vi "Ballard 1553 - Initialize.vi"(7 "RT Config Filepath":path, 8 "Error (in)":errorcluster, 9 "Compiled.Settings":T1 {"channels"."RTs"."Mode Codes"."Timestamp Channel Data Reference" format="%.0x"; "channels"."RTs"."subAddresses"."Timestamp Channel Data Reference" format="%.0x"; "channels"."RTs"."Status Channel Data Reference" format="%.0x"; "channels"."RTs"."Command Channels Refs" format="%.0x"; "channels"."BC"."Acyclic Frames Trigger Channels Refs" format="%.0x"; "channels"."BC"."Command Channels Refs" format="%.0x"; "channels"."BC"."messages"."Timestamp Channel Data Reference" format="%.0x"; "channels"."BC"."messages"."Status Channel Data Refs" format="%.0x"; "channels"."BC"."messages"."Words Item Refs" format="%.0x"}, 11 "Card Parameters (in)":T16) -> (0 "Error (out)":errorcluster, 3 "Card Parameters (out)":T16)   [LabVIEW 2019, in "Ballard MIL-1553 Engine.lvlib"]
doc: "Arinc-429 Board Initialization."
uses:
  Ballard MIL-1553 Engine.lvlib
  Controls/Card Parameters.ctl
  Shared/Controls and Global/Initialization Method.ctl
  Shared/Controls and Global/Compiled.Settings.ctl
  Shared/Controls and Global/RT Channel.ctl
  Shared/Controls and Global/RT BC.ctl
  <vilib>/NI VeriStand/Custom Device API/Custom Device Item Ref.ctl
  Shared/Controls and Global/RT Message.ctl
  Shared/Controls and Global/RT messageType.ctl
  Shared/Controls and Global/RT CWD1.ctl
  Shared/Controls and Global/RT CWD2.ctl
  <vilib>/NI VeriStand/Custom Device API/Data Reference.ctl
  <vilib>/NI VeriStand/Custom Device API/Block Data Reference.ctl
  Shared/Controls and Global/RT Remote Terminal.ctl
  Shared/Controls and Global/RT Remote Terminal_rtMode.ctl
  Shared/Controls and Global/RT Remote Terminal_RT subAddress.ctl
  Shared/Controls and Global/RT Remote Terminal_RT direction.ctl
  Shared/Controls and Global/RT Remote Terminal_RT Mode Code.ctl
  <instrlib>/BTICardLib/Private/Initialize By Card Number and Core Number.vi
  <instrlib>/BTICardLib/Private/Initialize By Slot Number and Core Number.vi
  <instrlib>/BTICardLib/Private/IO/Action-Status/Write External LED.vi
  <instrlib>/BTICardLib/Private/Configure All From XML.vi
  <instrlib>/BTI1553Lib/Private/Channel/Configure/Configure All From XML.vi
  <instrlib>/BTICardLib/BTICardLV.lvlib
  Shared/Ballard 1553 Shared.lvlib
  <instrlib>/BTI1553Lib/BTI1553LV.lvlib
  <vilib>/NI VeriStand/Custom Device Tools/Custom Device Utility Library/Custom Device Utility Library.lvlib
  <vilib>/NI VeriStand/Custom Device API/Custom Device API.lvlib
panel:
  out "Card Type":string
  out "Product String":string
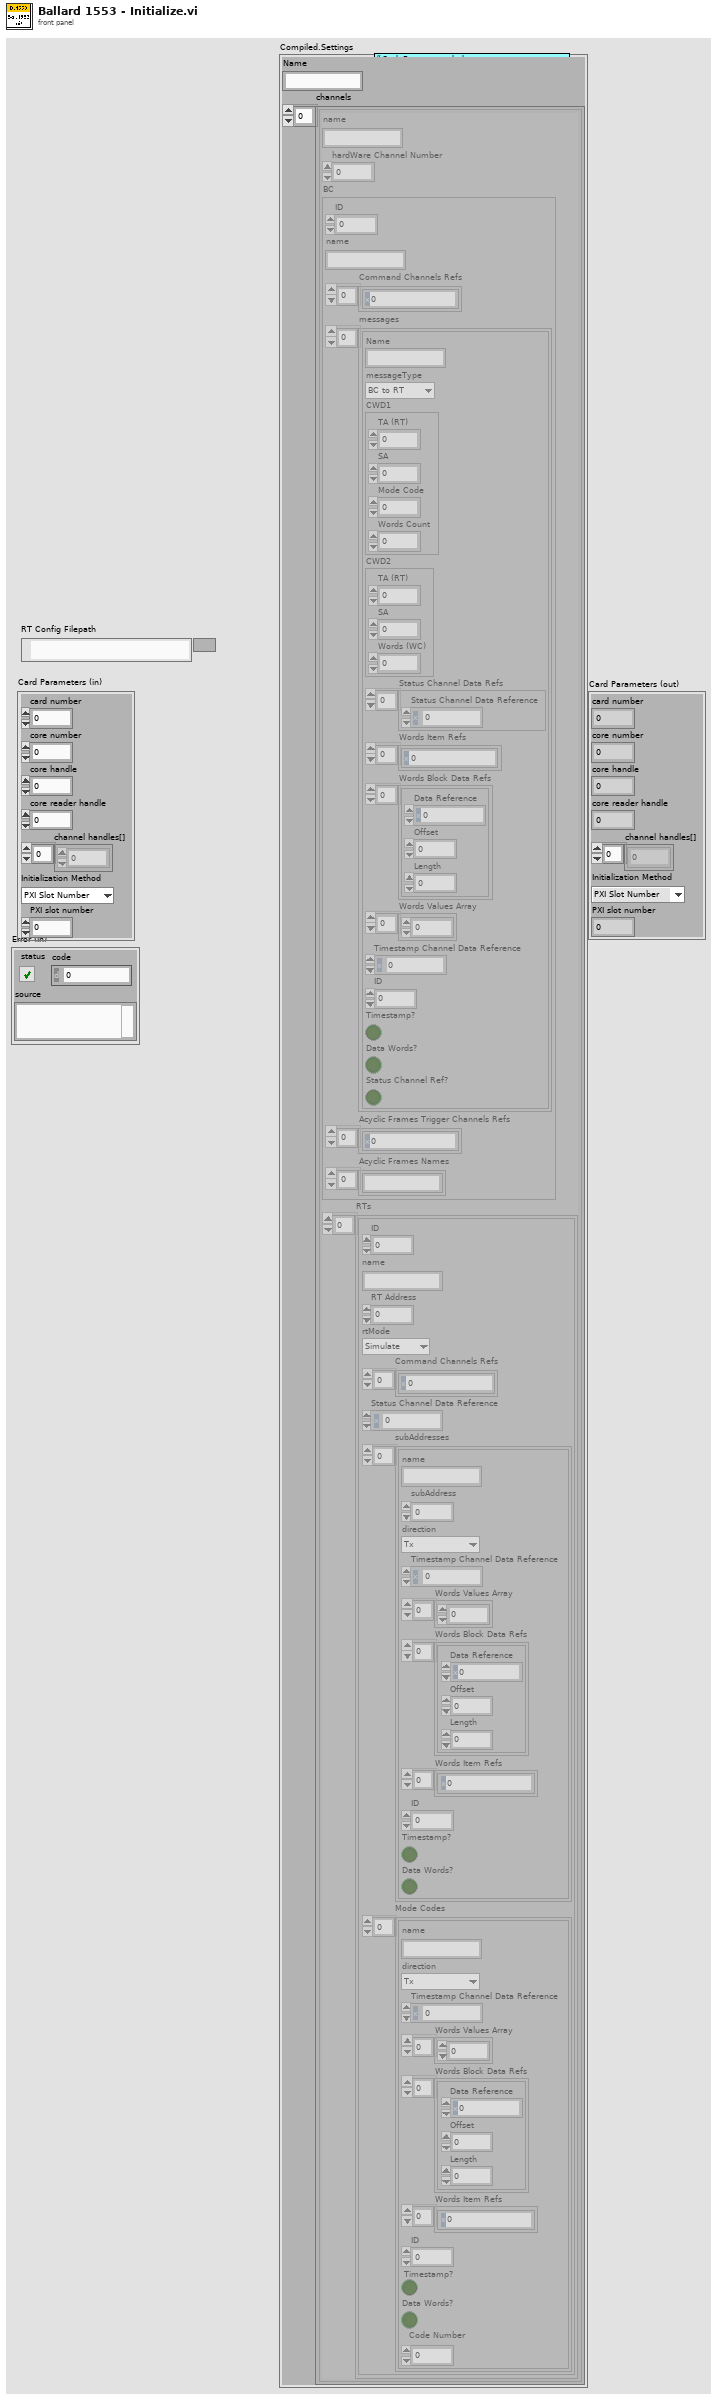
[diagram p1: front panel]
types:
  T1 = typedef "Ballard 1553 Shared.lvlib/Compiled.Settings.ctl" = cluster{"Name":string, "channels":T2[]}
  T2 = typedef "Ballard 1553 Shared.lvlib/RT Channel.ctl" = cluster{"name":string, "hardWare Channel Number":u16, "BC":T3, "RTs":T11[]}
  T3 = typedef "Ballard 1553 Shared.lvlib/RT BC.ctl" = cluster{"ID":i32, "name":string, "Command Channels Refs":T4[], "messages":T5[], "Acyclic Frames Trigger Channels Refs":T4[], "Acyclic Frames Names":string[]}
  T4 = typedef "Custom Device API.lvlib/Custom Device Item Ref.ctl" = u64
  T5 = typedef "Ballard 1553 Shared.lvlib/RT Message.ctl" = cluster{"Name":string, "messageType":T6, "CWD1":T7, "CWD2":T8, "Status Channel Data Refs":T9[], "Words Item Refs":T4[], "Words Block Data Refs":T10[], "Words Values Array":u16[], "Timestamp Channel Data Reference":T9, "ID":i32, "Timestamp?":bool, "Data Words?":bool, "Status Channel Ref?":bool}
  T6 = typedef "Ballard 1553 Shared.lvlib/RT messageType.ctl" = enum16{"BC to RT", "RT to BC", "RT to RT", "MC (Rx)", "MC (Tx)"}
  T7 = typedef "Ballard 1553 Shared.lvlib/RT CWD1.ctl" = cluster{"TA (RT)":i8, "SA":i8, "Mode Code":i8, "Words Count":i8}
  T8 = typedef "Ballard 1553 Shared.lvlib/RT CWD2.ctl" = cluster{"TA (RT)":i8, "SA":i8, "Words (WC)":i8}
  T9 = typedef "Custom Device API.lvlib/Data Reference.ctl" = i32
  T10 = typedef "Custom Device API.lvlib/Block Data Reference.ctl" = cluster{"Data Reference":T9, "Offset":u64, "Length":u64}
  T11 = typedef "Ballard 1553 Shared.lvlib/RT Remote Terminal.ctl" = cluster{"ID":i32, "name":string, "RT Address":i32, "rtMode":T12, "Command Channels Refs":T4[], "Status Channel Data Reference":T9, "subAddresses":T13[], "Mode Codes":T15[]}
  T12 = typedef "Ballard 1553 Shared.lvlib/RT Remote Terminal_rtMode.ctl" = enum16{"Simulate", "Monitor", "Disable"}
  T13 = typedef "Ballard 1553 Shared.lvlib/RT Remote Terminal_RT subAddress.ctl" = cluster{"name":string, "subAddress":i8, "direction":T14, "Timestamp Channel Data Reference":T9, "Words Values Array":u16[], "Words Block Data Refs":T10[], "Words Item Refs":T4[], "ID":i32, "Timestamp?":bool, "Data Words?":bool}
  T14 = typedef "Ballard 1553 Shared.lvlib/RT Remote Terminal_RT direction.ctl" = enum16{"Tx", "Rx"}
  T15 = typedef "Ballard 1553 Shared.lvlib/RT Remote Terminal_RT Mode Code.ctl" = cluster{"name":string, "direction":T14, "Timestamp Channel Data Reference":T9, "Words Values Array":u16[], "Words Block Data Refs":T10[], "Words Item Refs":T4[], "ID":i32, "Timestamp?":bool, "Data Words?":bool, "Code Number":i32}
  T16 = typedef "Ballard MIL-1553 Engine.lvlib/Card Parameters.ctl" = cluster{"card number":i32, "core number":i32, "core handle":u64, "core reader handle":u64, "channel handles[]":u64[], "Initialization Method":T17, "PXI slot number":i32}
  T17 = typedef "Ballard 1553 Shared.lvlib/Initialization Method.ctl" = enum16{"PXI Slot Number", "Card Number"}
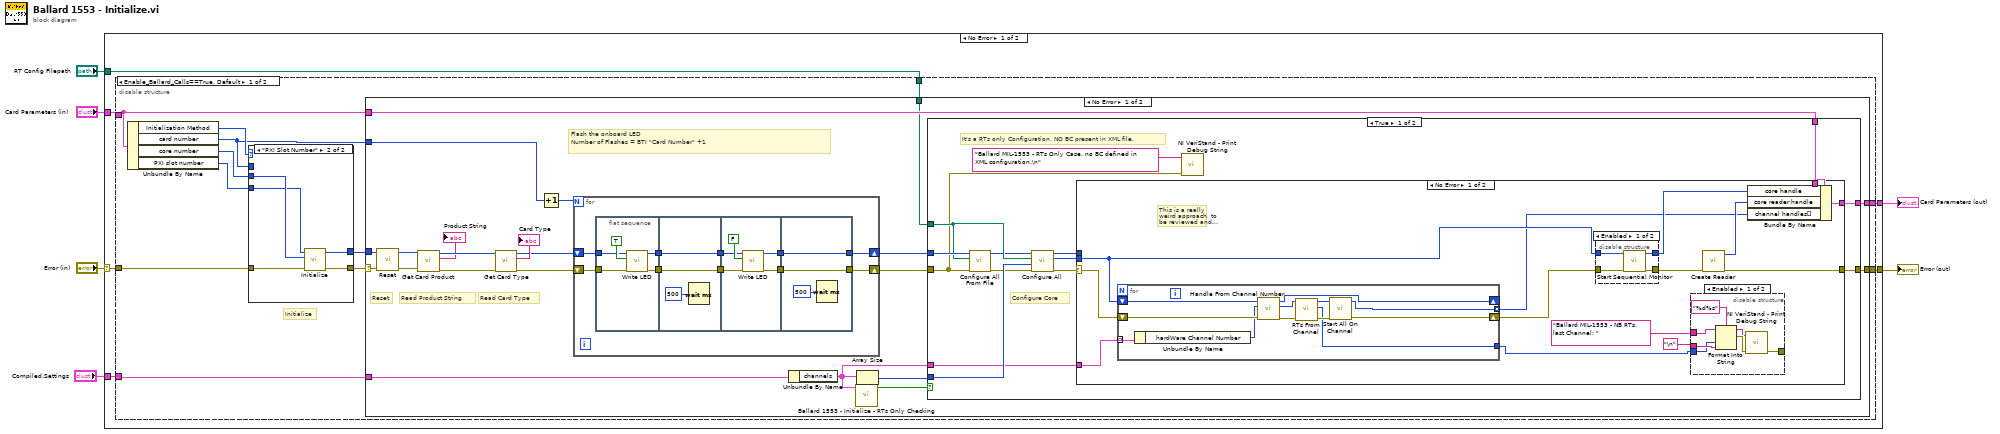
[diagram p0: block diagram]
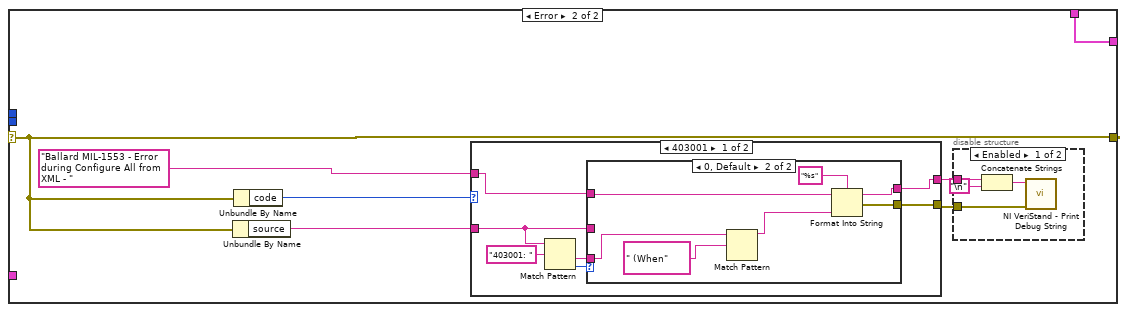
[diagram p4: hidden frame]
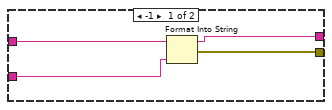
[diagram p6: hidden frame]
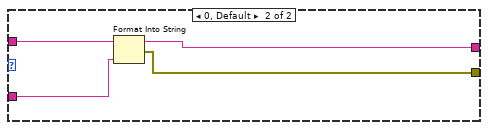
[diagram p7: hidden frame]
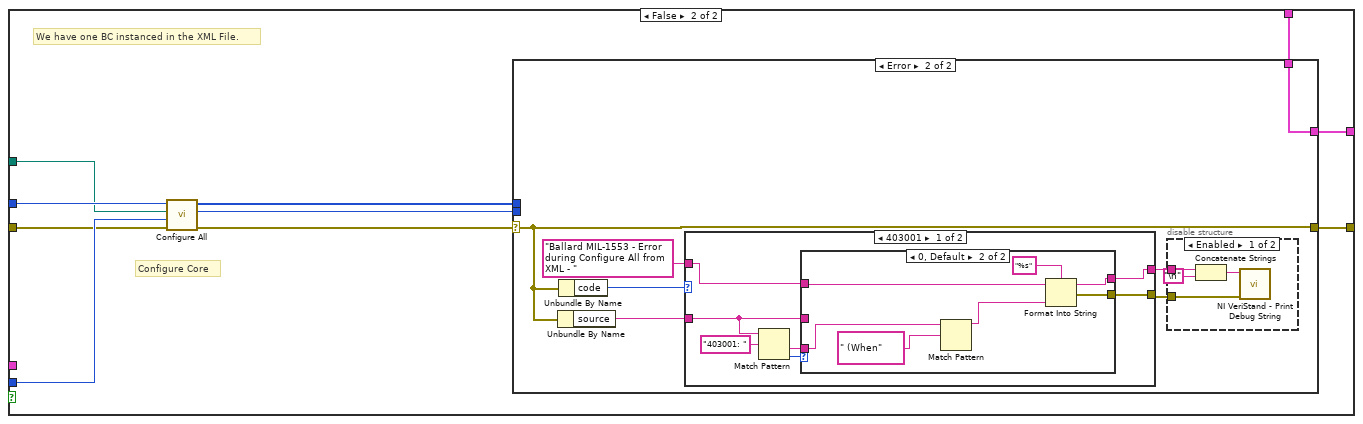
[diagram p8: hidden frame]
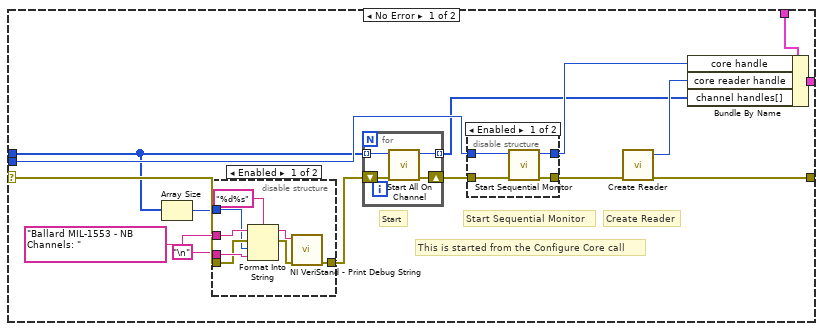
[diagram p9: hidden frame]
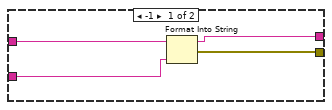
[diagram p13: hidden frame]
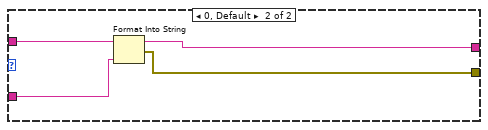
[diagram p14: hidden frame]
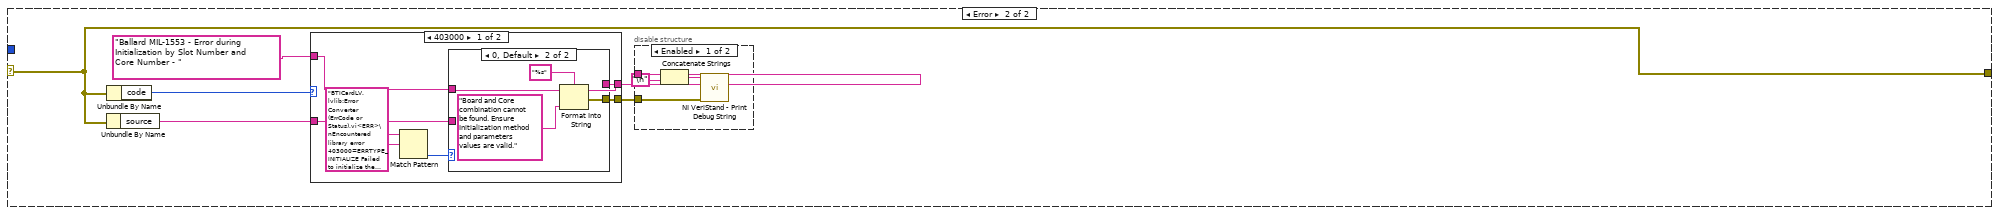
[diagram p15: hidden frame]
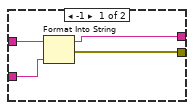
[diagram p17: hidden frame]
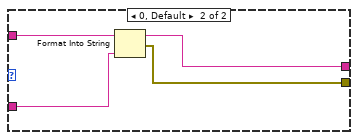
[diagram p18: hidden frame]
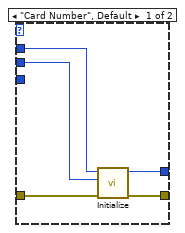
[diagram p19: hidden frame]
diagram:
  n1 = case shown="No Error" "Error (in)" {
    selector: "Error (in)" -> [w9 w279]
    tunnel: [w12 T16 {"card number"=0, "core number"=0, "core handle"=0, "core reader handle"=0, "channel handles[]"=[], "Initialization Method"=enum."PXI Slot Number", "PXI slot number"=0} ("Card Parameters (in)")] -> w6
    tunnel: "RT Config Filepath" -> [w11 _]
    tunnel: [w10 w279] -> w4
    tunnel: "Card Parameters (in)" -> [w8 _]
    tunnel: "Compiled.Settings" -> [w7 _]
    frame No Error {
      n2 = disable-structure shown="Enable_Ballard_Calls==True, Default" {
        disable-tunnel: [w23 w276] -> w12
        disable-tunnel: w11 -> [w15 _]
        disable-tunnel: [w14 w277] -> w10
        disable-tunnel: w9 -> [w22 w277]
        disable-tunnel: w8 -> [w21 w276]
        disable-tunnel: w7 -> [w16 _]
        frame condition #0 (active) {
          # "Initialize"
          n3 = Unbundle By Name(w21) -> ("Initialization Method"=w20:T17, "card number"=w19:i32, "core number"=w18:i32, "PXI slot number"=w17:i32)
          n4 = case shown="\"PXI Slot Number\"" w20 {
            tunnel: [w270 w275] -> w24
            tunnel: [w269 w274] -> w13
            tunnel: w19 -> [w268 _]
            tunnel: w22 -> [w267 w273]
            tunnel: w18 -> [w266 w272]
            tunnel: w17 -> [_ w271]
            frame "Card Number", Default {
              n5 = call-poly <instrlib>:"Initialize.vi"("error in (no error)"=w267, "core number"=w266, "card number"=w268) -> ("error out"=w269:errorcluster, "core handle out"=w270:u64)  [unwired: 7 in]
            }
            frame "PXI Slot Number" {
              n6 = call-poly <instrlib>:"Initialize.vi"("error in (no error)"=w273, "core number"=w272, "slot number"=w271) -> ("error out"=w274:errorcluster, "core handle out"=w275:u64)  [unwired: 7 in]
            }
          }
          n7 = case shown="No Error" w13 {
            selector: w13 -> [w29 w237]
            tunnel: w24 -> [w46 _]
            tunnel: [w45 _] -> w23
            tunnel: w21 -> [w35 _]
            tunnel: w19 -> [w34 _]
            tunnel: w16 -> [w33 _]
            tunnel: w15 -> [w27 _]
            tunnel: [w30 w237] -> w14
            frame No Error {
              # "Flash the onboard LED\nNumber of Flashes = BTI \"Card Number\" +1"
              # "Read Card Type"
              # "Read Product String"
              # "Reset"
              n8 = call <instrlib>:"Reset.vi"("error in (no error)"=w29, "core handle in"=w46) -> ("error out"=w39:errorcluster, "core handle out"=w40:u64)  [unwired: 8 in]
              n9 = call <instrlib>:"Get Card Product.vi"("error in (no error)"=w39, "core handle in"=w40) -> ("error out"=w43:errorcluster, "product string out"=→"Product String":string, "core handle out"=w44:u64)  [unwired: 7 in]
              n10 = call <instrlib>:"Get Card Type.vi"("error in (no error)"=w43, "core handle in"=w44) -> ("error out"=w37:errorcluster, "type string out"=→"Card Type":string, "core handle out"=w38:u64)  [unwired: 7 in]
              n11 = Increment(x=w34) -> (x+1=w36:i32)
              n12 = for {
                N: w36 -> [_]
                shift-right: [w212] -> w28
                shift-left: w38 -> [w214]
                shift-right: [w211] -> w31
                shift-left: w37 -> [w213]
                n13 = flat-sequence {
                  tunnel: [w224] -> w220
                  tunnel: [w223] -> w219
                  tunnel: w214 -> [w222]
                  tunnel: w213 -> [w221]
                  tunnel: [w227] -> w218
                  tunnel: w220 -> [w227]
                  tunnel: [w226] -> w217
                  tunnel: w219 -> [w226]
                  tunnel: w218 -> [w232]
                  tunnel: [w231] -> w216
                  tunnel: [w230] -> w215
                  tunnel: w217 -> [w229]
                  tunnel: [w235] -> w211
                  tunnel: w216 -> [w235]
                  tunnel: [w234] -> w212
                  tunnel: w215 -> [w234]
                  frame #0 {
                    n14 = call-poly <instrlib>:"Write LED.vi"("error in (no error)"=w221, "LED state"=TRUE, "core handle in"=w222) -> ("error out"=w224:errorcluster, "core handle out"=w223:u64)  [unwired: 7 in]
                  }
                  frame #1 {
                    n15 = Wait (ms)(milliseconds to wait=u32 500) -> ()  [unwired: 1 out]
                  }
                  frame #2 {
                    n16 = call-poly <instrlib>:"Write LED.vi"("error in (no error)"=w232, "LED state"=FALSE, "core handle in"=w229) -> ("error out"=w231:errorcluster, "core handle out"=w230:u64)  [unwired: 7 in]
                  }
                  frame #3 {
                    n17 = Wait (ms)(milliseconds to wait=u32 500) -> ()  [unwired: 1 out]
                  }
                }
              }
              n18 = Unbundle By Name(w33) -> ("channels"=w26:T2[])
              n19 = call "Ballard 1553 - Initialize - RTs Only Checking.vi"("channels"=w26) -> ("RTs Only?"=w25:bool)  [unwired: 10 in]
              n20 = Array Size(array=w26) -> (size(s)=w32:i32)
              n21 = case shown="True" w25 {
                tunnel: [w60 w143] -> w45
                tunnel: w35 -> [w59 w142]
                tunnel: w32 -> [w58 w141]
                tunnel: w31 -> [w47 w140]
                tunnel: [w57 w139] -> w30
                tunnel: w28 -> [w56 w138]
                tunnel: w27 -> [w55 w137]
                tunnel: w26 -> [w54 _]
                frame True {
                  # "It's a RTs only Configuration, NO BC present in XML file."
                  # "Configure Core"
                  n22 = call-poly <instrlib>:"Configure All From File.vi"("error in (no error)"=w47, "configuration file path"=w55, "core handle in"=w56) -> ("error out"=w49:errorcluster, "core handle out"=w50:u64)  [unwired: 7 in]
                  n23 = call-poly <instrlib>:"Configure All.vi"("error in (no error)"=w49, "channel handle array size in"=w58, "configuration file path"=w55, "core handle in"=w50) -> ("error out"=w51:errorcluster, "core handle out"=w53:u64, "channel handles out"=w52:u64[])  [unwired: 4 in, 1 out]
                  n24 = case shown="No Error" w51 {
                    selector: w51 -> [w66 w101]
                    tunnel: [w74 w102] -> w60
                    tunnel: w59 -> [w70 w102]
                    tunnel: w53 -> [w65 _]
                    tunnel: [w69 w101] -> w57
                    tunnel: w52 -> [_ _]
                    tunnel: w54 -> [w64 _]
                    frame No Error {
                      # "This is a really weird approach, to be reviewed and documented.\nIt comes from a trial and error,"
                      n25 = for {
                        tunnel: w64 -> [w84] mode=indexing
                        shift-right: [w78] -> w62
                        shift-left: w66 -> [w86]
                        shift-right: [w77] -> _
                        shift-left: w65 -> [w85]
                        tunnel: [w76] -> w63 mode=indexing
                        tunnel: [w75] -> w61
                        n26 = Unbundle By Name(w84) -> ("hardWare Channel Number"=w83:u16)
                        n27 = call <instrlib>:"Handle From Channel Number.vi"("error in (no error)"=w86, "channel number"=w83, "core handle in"=w85) -> ("error out"=w82:errorcluster, "channel handle out"=w81:u64, "core handle out"=w77:u64)  [unwired: 6 in]
                        n28 = call <instrlib>:"RTs From Channel.vi"("error in (no error)"=w82, "channel handle in"=w81) -> ("error out"=w79:errorcluster, "remote terminal count out"=w75:i32, "channel handle out"=w80:u64)  [unwired: 6 in, 1 out]
                        n29 = call <instrlib>:"Start All On Channel.vi"("error in (no error)"=w79, "channel handle in"=w80) -> ("error out"=w78:errorcluster, "channel handle out"=w76:u64)  [unwired: 8 in]
                      }
                      n30 = disable-structure shown="Enabled" {
                        disable-tunnel: w65 -> [w98 w100]
                        disable-tunnel: w62 -> [w97 w99]
                        disable-tunnel: [w96 w99] -> w71
                        disable-tunnel: [w95 w100] -> w72
                        frame Enabled {
                          n31 = call <instrlib>:"Start Sequential Monitor.vi"("error in (no error)"=w97, "core handle in"=w98) -> ("error out"=w96:errorcluster, "core handle out"=w95:u64)  [unwired: 8 in]
                        }
                        frame Disabled {
                        }
                      }
                      n32 = disable-structure shown="Enabled" {
                        disable-tunnel: "Ballard MIL-1553 - NB RTs, last Channel: " -> [w89 _]
                        disable-tunnel: w61 -> [w87 w94]
                        disable-tunnel: [w93 w94] -> _
                        disable-tunnel: "\n" -> [w92 _]
                        frame Enabled {
                          n33 = Format Into String(format string="%d%s", initial string=w89, w87, w92) -> (resulting string=w90:string, error out=w91:errorcluster)  [unwired: 1 in]
                          n34 = call <vilib>:"NI VeriStand - Print Debug String.vi"("error in (no error)"=w91, "Message"=w90) -> ("error out"=w93:errorcluster)  [unwired: 9 in]
                        }
                        frame Disabled {
                        }
                      }
                      n35 = call <instrlib>:"Create Reader.vi"("error in (no error)"=w71) -> ("error out"=w69:errorcluster, "core reader handle out"=w73:u64)  [unwired: 9 in]
                      n36 = Bundle By Name(cluster=w70, "core handle"=w72, "core reader handle"=w73, "channel handles[]"=w63) -> (w74:T16)
                    }
                    frame Error {
                      n37 = Unbundle By Name(w101) -> ("source"=w106:string)
                      n38 = Unbundle By Name(w101) -> ("code"=w107:i32)
                      n39 = case shown="403001" w107 {
                        tunnel: [w118 w131] -> w104
                        tunnel: [w117 w130] -> w105
                        tunnel: "Ballard MIL-1553 - Error during Configure All from XML - " ("String to write") -> [w115 w133]
                        tunnel: w106 -> [w116 w132]
                        frame 403001 {
                          n40 = Match Pattern(string=w116, regular expression="403001: ") -> (after substring=w112:string, offset past match=w114:i32)  [unwired: 1 in, 2 out]
                          n41 = case shown="0, Default" w114 {
                            tunnel: [w119 w129] -> w118
                            tunnel: [w120 w128] -> w117
                            tunnel: w116 -> [w121 _]
                            tunnel: w115 -> [w122 w127]
                            tunnel: w112 -> [_ w125]
                            frame -1 {
                              n42 = Format Into String(initial string=w122, w121) -> (resulting string=w119:string, error out=w120:errorcluster)  [unwired: 2 in]
                            }
                            frame 0, Default {
                              n43 = Match Pattern(string=w125, regular expression=" (When") -> (before substring=w124:string)  [unwired: 1 in, 3 out]
                              n44 = Format Into String(format string="%s", initial string=w127, w124) -> (resulting string=w129:string, error out=w128:errorcluster)  [unwired: 1 in]
                            }
                          }
                        }
                        frame 0, Default {
                          n45 = Format Into String(initial string=w133, w132) -> (resulting string=w131:string, error out=w130:errorcluster)  [unwired: 2 in]
                        }
                      }
                      n46 = disable-structure shown="Enabled" {
                        disable-tunnel: w105 -> [w109 _]
                        disable-tunnel: w104 -> [w108 _]
                        frame Enabled {
                          n47 = Concatenate Strings(w108, "\n") -> (w110:string)
                          n48 = call <vilib>:"NI VeriStand - Print Debug String.vi"("error in (no error)"=w109, "Message"=w110) -> ()  [unwired: 9 in, 1 out]
                        }
                        frame Disabled {
                        }
                      }
                    }
                  }
                  n49 = call <vilib>:"NI VeriStand - Print Debug String.vi"("error in (no error)"=w47, "Message"="Ballard MIL-1553 - RTs Only Case, no BC defined in XML configuration.\n") -> ()  [unwired: 9 in, 1 out]
                }
                frame False {
                  # "We have one BC instanced in the XML File."
                  # "Configure Core"
                  n50 = call-poly <instrlib>:"Configure All.vi"("error in (no error)"=w140, "channel handle array size in"=w141, "configuration file path"=w137, "core handle in"=w138) -> ("error out"=w134:errorcluster, "core handle out"=w136:u64, "channel handles out"=w135:u64[])  [unwired: 4 in, 1 out]
                  n51 = case shown="Error" w134 {
                    selector: w134 -> [w148 w178]
                    tunnel: [w158 w179] -> w143
                    tunnel: w142 -> [w154 w179]
                    tunnel: w136 -> [w152 _]
                    tunnel: [w151 w178] -> w139
                    tunnel: w135 -> [w145 _]
                    frame No Error {
                      # "This is started from the Configure Core call"
                      # "Start"
                      # "Start Sequential Monitor"
                      # "Create Reader"
                      n52 = Array Size(array=w145) -> (size(s)=w144:i32)
                      n53 = disable-structure shown="Enabled" {
                        disable-tunnel: "Ballard MIL-1553 - NB Channels: " -> [w161 _]
                        disable-tunnel: w148 -> [w164 w167]
                        disable-tunnel: [w166 w167] -> w147
                        disable-tunnel: "\n" -> [w165 _]
                        disable-tunnel: w144 -> [w160 _]
                        frame Enabled {
                          n54 = Format Into String(format string="%d%s", initial string=w161, error in=w164, w160, w165) -> (resulting string=w162:string, error out=w163:errorcluster)
                          n55 = call <vilib>:"NI VeriStand - Print Debug String.vi"("error in (no error)"=w163, "Message"=w162) -> ("error out"=w166:errorcluster)  [unwired: 9 in]
                        }
                        frame Disabled {
                        }
                      }
                      n56 = for {
                        shift-right: [w170] -> w153
                        shift-left: w147 -> [w171]
                        tunnel: w145 -> [w169] mode=indexing
                        tunnel: [w168] -> w150 mode=indexing
                        n57 = call <instrlib>:"Start All On Channel.vi"("error in (no error)"=w171, "channel handle in"=w169) -> ("error out"=w170:errorcluster, "channel handle out"=w168:u64)  [unwired: 8 in]
                      }
                      n58 = disable-structure shown="Enabled" {
                        disable-tunnel: w152 -> [w175 w177]
                        disable-tunnel: w153 -> [w174 w176]
                        disable-tunnel: [w173 w176] -> w155
                        disable-tunnel: [w172 w177] -> w156
                        frame Enabled {
                          n59 = call <instrlib>:"Start Sequential Monitor.vi"("error in (no error)"=w174, "core handle in"=w175) -> ("error out"=w173:errorcluster, "core handle out"=w172:u64)  [unwired: 8 in]
                        }
                        frame Disabled {
                        }
                      }
                      n60 = call <instrlib>:"Create Reader.vi"("error in (no error)"=w155) -> ("error out"=w151:errorcluster, "core reader handle out"=w157:u64)  [unwired: 9 in]
                      n61 = Bundle By Name(cluster=w154, "core handle"=w156, "core reader handle"=w157, "channel handles[]"=w150) -> (w158:T16)
                    }
                    frame Error {
                      n62 = Unbundle By Name(w178) -> ("source"=w183:string)
                      n63 = Unbundle By Name(w178) -> ("code"=w184:i32)
                      n64 = case shown="403001" w184 {
                        tunnel: [w195 w208] -> w181
                        tunnel: [w194 w207] -> w182
                        tunnel: "Ballard MIL-1553 - Error during Configure All from XML - " ("String to write") -> [w192 w210]
                        tunnel: w183 -> [w193 w209]
                        frame 403001 {
                          n65 = Match Pattern(string=w193, regular expression="403001: ") -> (after substring=w189:string, offset past match=w191:i32)  [unwired: 1 in, 2 out]
                          n66 = case shown="0, Default" w191 {
                            tunnel: [w196 w206] -> w195
                            tunnel: [w197 w205] -> w194
                            tunnel: w193 -> [w198 _]
                            tunnel: w192 -> [w199 w204]
                            tunnel: w189 -> [_ w202]
                            frame -1 {
                              n67 = Format Into String(initial string=w199, w198) -> (resulting string=w196:string, error out=w197:errorcluster)  [unwired: 2 in]
                            }
                            frame 0, Default {
                              n68 = Match Pattern(string=w202, regular expression=" (When") -> (before substring=w201:string)  [unwired: 1 in, 3 out]
                              n69 = Format Into String(format string="%s", initial string=w204, w201) -> (resulting string=w206:string, error out=w205:errorcluster)  [unwired: 1 in]
                            }
                          }
                        }
                        frame 0, Default {
                          n70 = Format Into String(initial string=w210, w209) -> (resulting string=w208:string, error out=w207:errorcluster)  [unwired: 2 in]
                        }
                      }
                      n71 = disable-structure shown="Enabled" {
                        disable-tunnel: w182 -> [w186 _]
                        disable-tunnel: w181 -> [w185 _]
                        frame Enabled {
                          n72 = Concatenate Strings(w185, "\n") -> (w187:string)
                          n73 = call <vilib>:"NI VeriStand - Print Debug String.vi"("error in (no error)"=w186, "Message"=w187) -> ()  [unwired: 9 in, 1 out]
                        }
                        frame Disabled {
                        }
                      }
                    }
                  }
                }
              }
            }
            frame Error {
              n74 = Unbundle By Name(w237) -> ("source"=w240:string)
              n75 = Unbundle By Name(w237) -> ("code"=w239:i32)
              n76 = case shown="403000" w239 {
                tunnel: [w252 w263] -> w242
                tunnel: [w251 w262] -> w241
                tunnel: "Ballard MIL-1553 - Error during Initialization by Slot Number and Core Number - " ("String to write") -> [w247 w265]
                tunnel: w240 -> [w248 w264]
                frame 403000 {
                  n77 = Match Pattern(string=w248, regular expression="BTICardLV.lvlib:Error Converter (ErrCode or Status).vi<ERR>\nEncountered library error 403000=ERRTYPE_INITIALIZE Failed to initialize the card or core (LabVIEW Library)\nDebug Info: No matching slot number was found in BTICardLV_InitializeBySlotNumber.") -> (offset past match=w249:i32)  [unwired: 1 in, 3 out]
                  n78 = case shown="0, Default" w249 {
                    tunnel: [w253 w261] -> w252
                    tunnel: [w254 w260] -> w251
                    tunnel: w248 -> [w255 _]
                    tunnel: w247 -> [w256 w259]
                    frame -1 {
                      n79 = Format Into String(initial string=w256, w255) -> (resulting string=w253:string, error out=w254:errorcluster)  [unwired: 2 in]
                    }
                    frame 0, Default {
                      n80 = Format Into String(format string="%s", initial string=w259, "Board and Core combination cannot be found. Ensure Initialization method and parameters values are valid.") -> (resulting string=w261:string, error out=w260:errorcluster)  [unwired: 1 in]
                    }
                  }
                }
                frame 0, Default {
                  n81 = Format Into String(initial string=w265, w264) -> (resulting string=w263:string, error out=w262:errorcluster)  [unwired: 2 in]
                }
              }
              n82 = disable-structure shown="Enabled" {
                disable-tunnel: w241 -> [w244 _]
                disable-tunnel: w242 -> [w243 _]
                frame Enabled {
                  n83 = Concatenate Strings(w243, "\n") -> (w245:string)
                  n84 = call <vilib>:"NI VeriStand - Print Debug String.vi"("error in (no error)"=w244, "Message"=w245) -> ()  [unwired: 9 in, 1 out]
                }
                frame Disabled {
                }
              }
            }
          }
        }
        frame condition #1 {
        }
      }
    }
    frame Error {
    }
  }
  "Error (out)" <- w4
  "Card Parameters (out)" <- w6
